vi "IMUtoNormalGyro.vi"(9 "IMU Data":T1) -> (0 "Yaw":dbl, 1 "Roll":dbl, 2 "Pitch":dbl, 3 "IMU Data Out":cluster{"Pitch":dbl, "Roll":dbl, "Yaw":dbl})   [LabVIEW 2015]
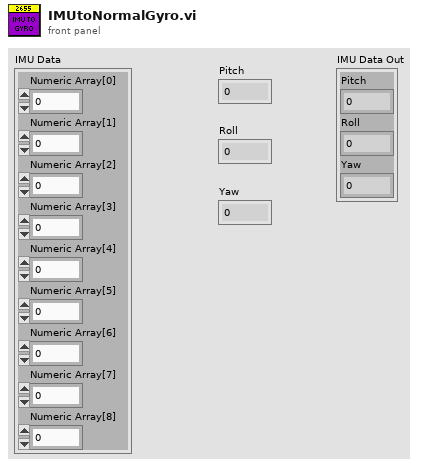
[diagram p1: front panel]
types:
  T1 = cluster{"Numeric Array[0]":dbl, "Numeric Array[1]":dbl, "Numeric Array[2]":dbl, "Numeric Array[3]":dbl, "Numeric Array[4]":dbl, "Numeric Array[5]":dbl, "Numeric Array[6]":dbl, "Numeric Array[7]":dbl, "Numeric Array[8]":dbl}
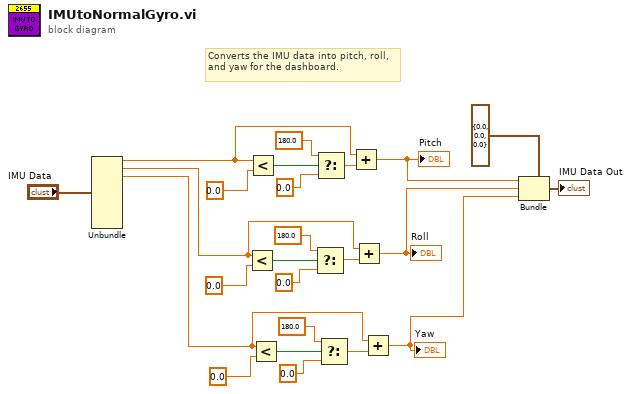
[diagram p0: block diagram]
diagram:
  # "Converts the IMU data into pitch, roll, and yaw for the dashboard."
  n1 = Unbundle("IMU Data") -> ("Numeric Array[0]"=w8:dbl, "Numeric Array[1]"=w5:dbl, "Numeric Array[2]"=w1:dbl)  [unwired: 6 out]
  n2 = Less?(x=w5, y=0.0) -> (x < y?=w20:bool)
  n3 = Less?(x=w8, y=0.0) -> (x < y?=w24:bool)
  n4 = Less?(x=w1, y=0.0) -> (x < y?=w16:bool)
  n5 = Select(t=180.0, s=w20, f=0.0) -> (s? t:f=w6:dbl)
  n6 = Select(t=180.0, s=w24, f=0.0) -> (s? t:f=w9:dbl)
  n7 = Select(t=180.0, s=w16, f=0.0) -> (s? t:f=w2:dbl)
  n8 = Add(x=w8, y=w9) -> (x+y=w7:dbl)
  "Pitch" <- w7
  n9 = Add(x=w5, y=w6) -> (x+y=w4:dbl)
  "Roll" <- w4
  n10 = Add(x=w1, y=w2) -> (x+y=w3:dbl)
  "Yaw" <- w3
  n11 = Bundle(cluster=cluster{"Pitch":dbl, "Roll":dbl, "Yaw":dbl} {"Pitch"=0.0, "Roll"=0.0, "Yaw"=0.0} ("IMU AHRS"), "Pitch"=w7, "Roll"=w4, "Yaw"=w3) -> (→"IMU Data Out":cluster{"Pitch":dbl, "Roll":dbl, "Yaw":dbl})
